vi "Get Distance Order.vi"(8 "error in (no error)":errorcluster, 11 "KD Tree in":refnum<class "KD Tree.lvclass">) -> (0 "error out":errorcluster, 2 "Minkowski Distance Order":i32, 3 "KD Tree out":refnum<class "KD Tree.lvclass">)   [LabVIEW 2020, in "KD Tree.lvlib" / "KD Tree.lvclass"]
uses:
  KD Tree.lvclass
  KD Tree.lvlib
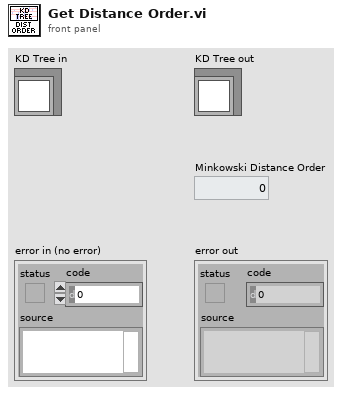
[diagram p1: front panel]
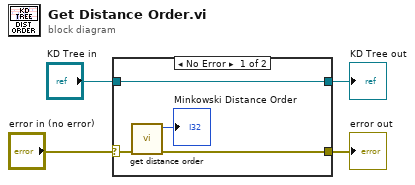
[diagram p0: block diagram]
diagram:
  n1 = case shown="No Error" "error in (no error)" {
    selector: "error in (no error)" -> [w7 w10]
    tunnel: [w6 w10] -> w3
    tunnel: [w8 w9] -> w1
    tunnel: "KD Tree in" -> [w8 w9]
    frame No Error {
      n2 = call "get distance order.vi"("error in (no error)"=w7) -> ("error out"=w6:errorcluster, "Minkowski Distance Order"=→"Minkowski Distance Order":i32)  [unwired: 9 in]
    }
    frame Error {
    }
  }
  "error out" <- w3
  "KD Tree out" <- w1
